vi "changeMode.vi"(8 "error in (no error)":errorcluster, 10 "ElectrometerController in":refnum<class "ElectrometerController.lvclass">, 11 "State in":refnum<class "ElectrometerState.lvclass">) -> (0 "error out":errorcluster, 2 "ElectrometerController out":refnum<class "ElectrometerController.lvclass">, 3 "State out":refnum<class "ElectrometerState.lvclass">)   [LabVIEW 2016, in "ElectrometerState.lvclass"]
uses:
  ElectrometerState.lvclass
  ElectrometerController/ElectrometerController.lvclass
  ts_electrometeruserevents/Typedefs/RejectedCommand.ctl
  ts_electrometeruserevents/Typedefs/CommandValue.ctl
  ts_electrometeruserevents/Typedefs/StateValue.ctl
  ts_electrometeruserevents/Typedefs/ElectrometerTypedefs.lvlib
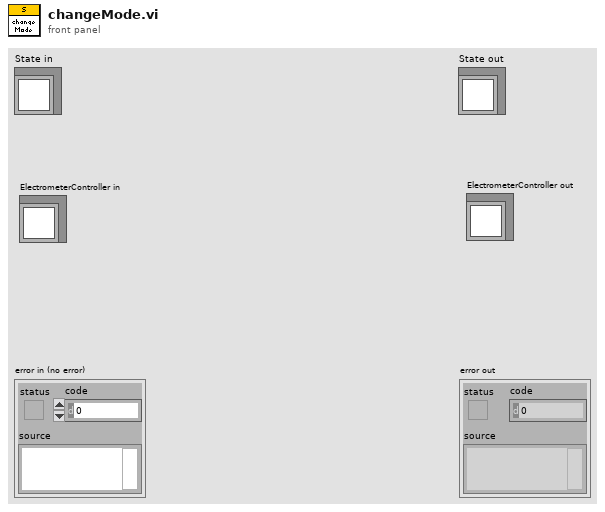
[diagram p1: front panel]
types:
  T1 = typedef "ElectrometerTypedefs.lvlib/RejectedCommand.ctl" = cluster{"CommandValue":T2, "StateValue":T3, "Time Stamp":dbl}
  T2 = typedef "ElectrometerTypedefs.lvlib/CommandValue.ctl" = enum16{"ClearError", "Disable", "Enable", "Exit", "GoToStandby", "OnHeartbeat", "OnIncomingMessagingError", "OnInterrupt", "Start", "SetDigitalFilter", "StartScan", "StartScanDt", "StartScanReachIntensity", "StopScan", "SetIntegrationTime", "PerformZeroCalib", "SetRange", "SetMode", "Power"}
  T3 = typedef "ElectrometerTypedefs.lvlib/StateValue.ctl" = enum16{"", "DisabledState", "EnabledState", "FaultState", "OffState", "StandbyState", "SetDurationReadingState", "ConfiguringState", "ReadyState", "ManualReadingState", "UntilIntentisyReadingState"}
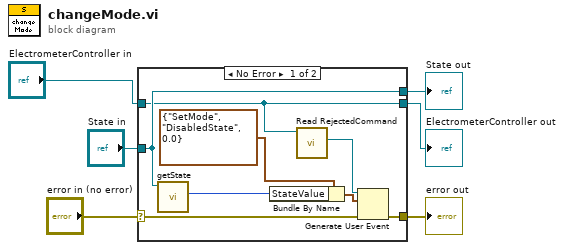
[diagram p0: block diagram]
diagram:
  n1 = case shown="No Error" "error in (no error)" {
    selector: "error in (no error)" -> [w11 w17]
    tunnel: [w10 w17] -> w5
    tunnel: [w9 w16] -> w3
    tunnel: "State in" -> [w9 w16]
    tunnel: "ElectrometerController in" -> [w8 w15]
    tunnel: [w8 w15] -> w1
    frame No Error {
      n2 = call-dynamic "getState.vi"("State in"=w9) -> ("StateValue"=w12:T3)  [unwired: 8 in, 2 out]
      n3 = Bundle By Name(cluster=T1 {"CommandValue"=enum."SetMode", "StateValue"=enum."DisabledState", "Time Stamp"=0.0} ("event data"), "StateValue"=w12) -> (w13:T1)
      n4 = call-dynamic "Read RejectedCommand.vi"("ElectrometerController in"=w8) -> ("RejectedCommand"=w7:refnum<user-event>)  [unwired: 8 in, 2 out]
      n5 = Generate User Event(user event=w7, event data cluster=w13, error in=w11) -> (error out=w10:errorcluster)  [unwired: 1 in, 1 out]
    }
    frame Error {
    }
  }
  "error out" <- w5
  "State out" <- w3
  "ElectrometerController out" <- w1
